vi "波形倍数.vi"(2 "时域波形图":waveform(dbl)[](graph), 6 "数值":dbl, 7 "数值 5":dbl, 8 "数值 2":dbl, 9 "数值 6":dbl, 10 "数值 3":dbl, 11 "数值 7":dbl, 12 "数值 4":dbl, 13 "数值 8":dbl) -> (16 "时域波形图 2":waveform(dbl)[](graph))   [LabVIEW 2014]
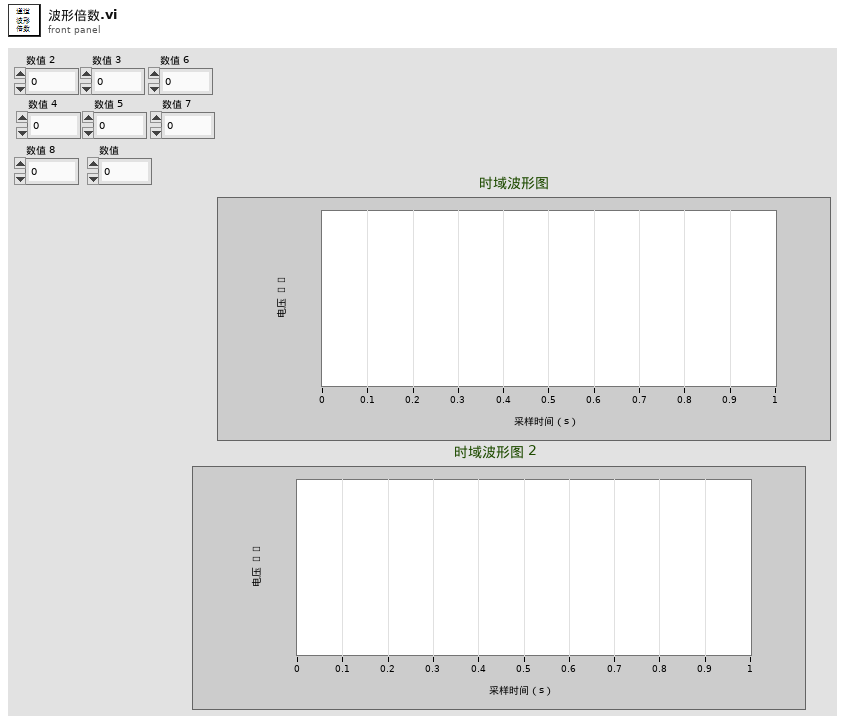
[diagram p1: front panel]
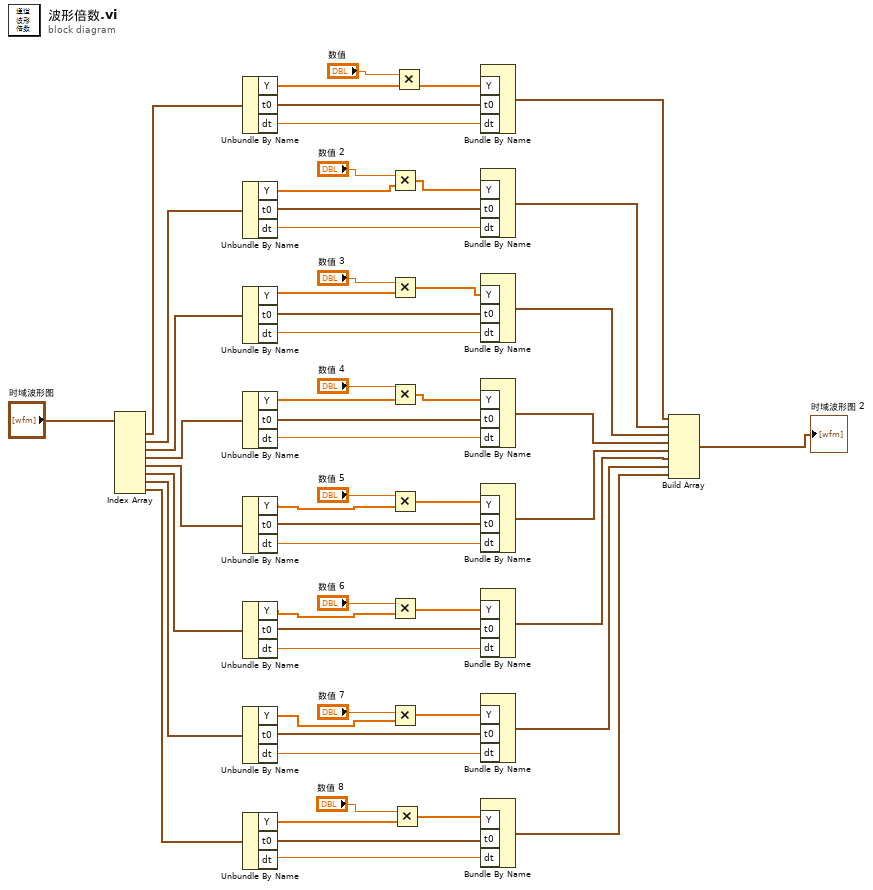
[diagram p0: block diagram]
diagram:
  n1 = Index Array(array="时域波形图") -> (element #1=w57:waveform(dbl), element #2=w56:waveform(dbl), element #3=w55:waveform(dbl), element #4=w54:waveform(dbl), element #5=w53:waveform(dbl), element #6=w52:waveform(dbl), element #7=w51:waveform(dbl), element #8=w50:waveform(dbl))  [unwired: 8 in]
  n2 = Unbundle By Name(w57) -> ("Y"=w48:dbl[], "t0"=w32:timestamp, "dt"=w31:dbl)
  n3 = Unbundle By Name(w56) -> ("Y"=w46:dbl[], "t0"=w26:timestamp, "dt"=w25:dbl)
  n4 = Unbundle By Name(w55) -> ("Y"=w44:dbl[], "t0"=w23:timestamp, "dt"=w22:dbl)
  n5 = Unbundle By Name(w54) -> ("Y"=w42:dbl[], "t0"=w20:timestamp, "dt"=w19:dbl)
  n6 = Unbundle By Name(w53) -> ("Y"=w40:dbl[], "t0"=w17:timestamp, "dt"=w16:dbl)
  n7 = Unbundle By Name(w52) -> ("Y"=w38:dbl[], "t0"=w14:timestamp, "dt"=w13:dbl)
  n8 = Unbundle By Name(w51) -> ("Y"=w36:dbl[], "t0"=w11:timestamp, "dt"=w10:dbl)
  n9 = Unbundle By Name(w50) -> ("Y"=w34:dbl[], "t0"=w29:timestamp, "dt"=w28:dbl)
  n10 = Multiply(x="数值 2", y=w46) -> (x*y=w27:dbl[])
  n11 = Multiply(x="数值 3", y=w44) -> (x*y=w24:dbl[])
  n12 = Multiply(x="数值 4", y=w42) -> (x*y=w21:dbl[])
  n13 = Multiply(x="数值 5", y=w40) -> (x*y=w18:dbl[])
  n14 = Multiply(x="数值 6", y=w38) -> (x*y=w15:dbl[])
  n15 = Multiply(x="数值 7", y=w36) -> (x*y=w12:dbl[])
  n16 = Multiply(x="数值 8", y=w34) -> (x*y=w30:dbl[])
  n17 = Multiply(x="数值", y=w48) -> (x*y=w33:dbl[])
  n18 = Bundle By Name("Y"=w33, "t0"=w32, "dt"=w31) -> (w9:waveform(dbl))  [unwired: 1 in]
  n19 = Bundle By Name("Y"=w27, "t0"=w26, "dt"=w25) -> (w8:waveform(dbl))  [unwired: 1 in]
  n20 = Bundle By Name("Y"=w24, "t0"=w23, "dt"=w22) -> (w7:waveform(dbl))  [unwired: 1 in]
  n21 = Bundle By Name("Y"=w21, "t0"=w20, "dt"=w19) -> (w6:waveform(dbl))  [unwired: 1 in]
  n22 = Bundle By Name("Y"=w18, "t0"=w17, "dt"=w16) -> (w5:waveform(dbl))  [unwired: 1 in]
  n23 = Bundle By Name("Y"=w15, "t0"=w14, "dt"=w13) -> (w4:waveform(dbl))  [unwired: 1 in]
  n24 = Bundle By Name("Y"=w12, "t0"=w11, "dt"=w10) -> (w3:waveform(dbl))  [unwired: 1 in]
  n25 = Bundle By Name("Y"=w30, "t0"=w29, "dt"=w28) -> (w2:waveform(dbl))  [unwired: 1 in]
  n26 = Build Array(w9, w8, w7, w6, w5, w4, w3, w2) -> (→"时域波形图 2":waveform(dbl)[])
